vi "Escape.vi"(10 "Escape Equal Sign":bool=TRUE, 11 "String in":string) -> (3 "String out":string)   [LabVIEW 2018]
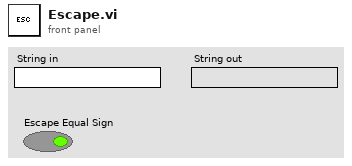
[diagram p1: front panel]
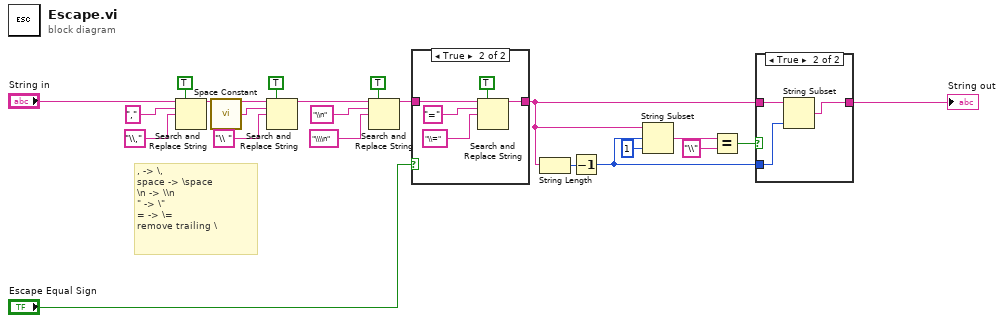
[diagram p0: block diagram]
diagram:
  # ", -> \\,\nspace -> \\space\n\\n -> \\\\n\n\" -> \\\"\n= -> \\=\nremove trailing \\"
  n1 = Search and Replace String(replace all?=TRUE ("replace all? (F)"), input string="String in", search string="," ("replace string (\"\")"), replace string="\\," ("replace string (\"\")")) -> (result string=w8:string)  [unwired: 4 in, 3 out]
  n2 = call <vilib>:"Space Constant.vi"() -> ("String"=w7:string)
  n3 = Search and Replace String(replace all?=TRUE ("replace all? (F)"), input string=w8, search string=w7, replace string="\\ " ("replace string (\"\")")) -> (result string=w12:string)  [unwired: 4 in, 3 out]
  n4 = Search and Replace String(replace all?=TRUE ("replace all? (F)"), input string=w12, search string="\\n" ("replace string (\"\")"), replace string="\\\\n" ("replace string (\"\")")) -> (result string=w13:string)  [unwired: 4 in, 3 out]
  n5 = case shown="True" "Escape Equal Sign" {
    tunnel: w13 -> [w23 w25]
    tunnel: [w23 w24] -> w20
    frame False {
    }
    frame True {
      n6 = Search and Replace String(replace all?=TRUE ("replace all? (F)"), input string=w25, search string="=" ("replace string (\"\")"), replace string="\\=" ("replace string (\"\")")) -> (result string=w24:string)  [unwired: 4 in, 3 out]
    }
  }
  n7 = String Length(string=w20) -> (length=w14:i32)
  n8 = Decrement(x=w14) -> (x-1=w21:i32)
  n9 = String Subset(string=w20, offset (0)=w21, length (rest)=1 ("length (rest)")) -> (substring=w17:string)
  n10 = Equal?(x=w17, y="\\") -> (x = y?=w19:bool)
  n11 = case shown="True" w19 {
    tunnel: w20 -> [w29 w32]
    tunnel: w21 -> [_ w31]
    tunnel: [w29 w30] -> w22
    frame False {
    }
    frame True {
      n12 = String Subset(string=w32, length (rest)=w31) -> (substring=w30:string)  [unwired: 1 in]
    }
  }
  "String out" <- w22
